vi "PrepareHWI.vi"(8 "error in (no error)":errorcluster, 9 "Master Device in":refnum<class "Master Device.lvclass">, 10 "Current Variables":T1[](array[typedef]), 11 "Master Device in":refnum<class "Master Device.lvclass">) -> (0 "error out":errorcluster, 2 "Master Device out":refnum<class "Master Device.lvclass">, 3 "Master Device out":refnum<class "Master Device.lvclass">)   [LabVIEW 2013, in "Master Device.lvclass"]
uses:
  Master Device.lvclass
  TypeDefs/Active procedure variables.ctl
  Device/Device.lvclass
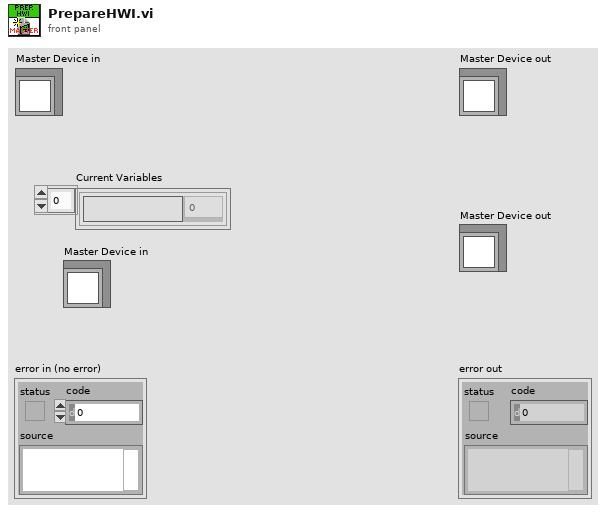
[diagram p1: front panel]
types:
  T1 = typedef "Active procedure variables.ctl" = cluster{"Procedure variable":string, "Value":dbl}
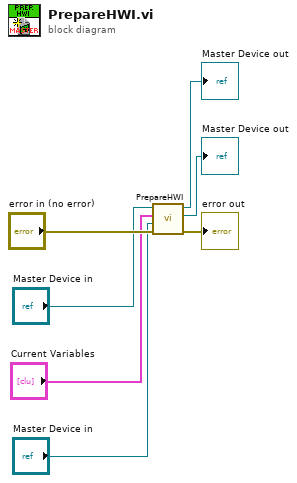
[diagram p0: block diagram]
diagram:
  n1 = call-parent "PrepareHWI.vi"("error in (no error)"="error in (no error)", "Master Device in"="Master Device in", "Current Variables"="Current Variables", "Device in"="Master Device in") -> ("error out"=→"error out":errorcluster, "Master Device out"=→"Master Device out":refnum<class "Master Device.lvclass">, "Device out"=→"Master Device out":refnum<class "Master Device.lvclass">)  [unwired: 5 in]
